vi "Set Time Settings.vi"(8 "error in":errorcluster, 11 "DateTime":T1) -> (0 "error out":errorcluster)   [LabVIEW 2016, in "RT Management.lvlib" / "RT Management.lvclass"]
uses:
  RT Management.lvclass
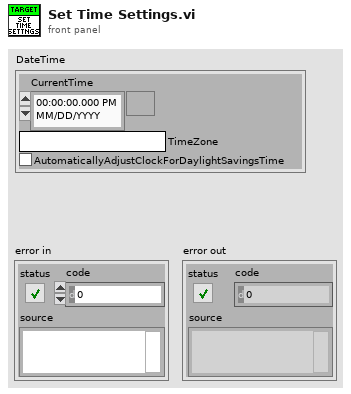
[diagram p1: front panel]
types:
  T1 = cluster{"CurrentTime":timestamp, "TimeZone":string, "AutomaticallyAdjustClockForDaylightSavingsTime":bool}
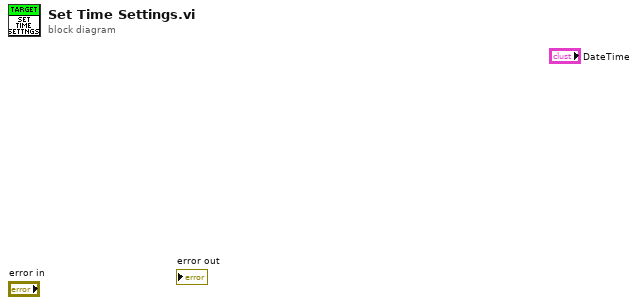
[diagram p0: block diagram]
diagram:
